vi "WILT Process Cycle Data.vi"(7 "WILT Summary Input":T1[](array[typedef]), 9 "Inverter File Headers":string[](array[string]), 10 "File Locations":T2[](array[typedef]), 11 "New File":bool[](array[boolean])) -> (2 "Units to Process":bool[](array[boolean]), 3 "WILT Summary Output":T1[](array[typedef]))   [LabVIEW 2016]
uses:
  Utility/Save File/File Setup (Public)/Type Definition/Save File DOE File Path Control.ctl
  Utility/Save File/File Setup (Public)/Type Definition/Save File DOE Data Save Filepaths.ctl
  Type Definitions/WILT Summary Data.ctl
  Utility/Save File/File Setup.lvlib
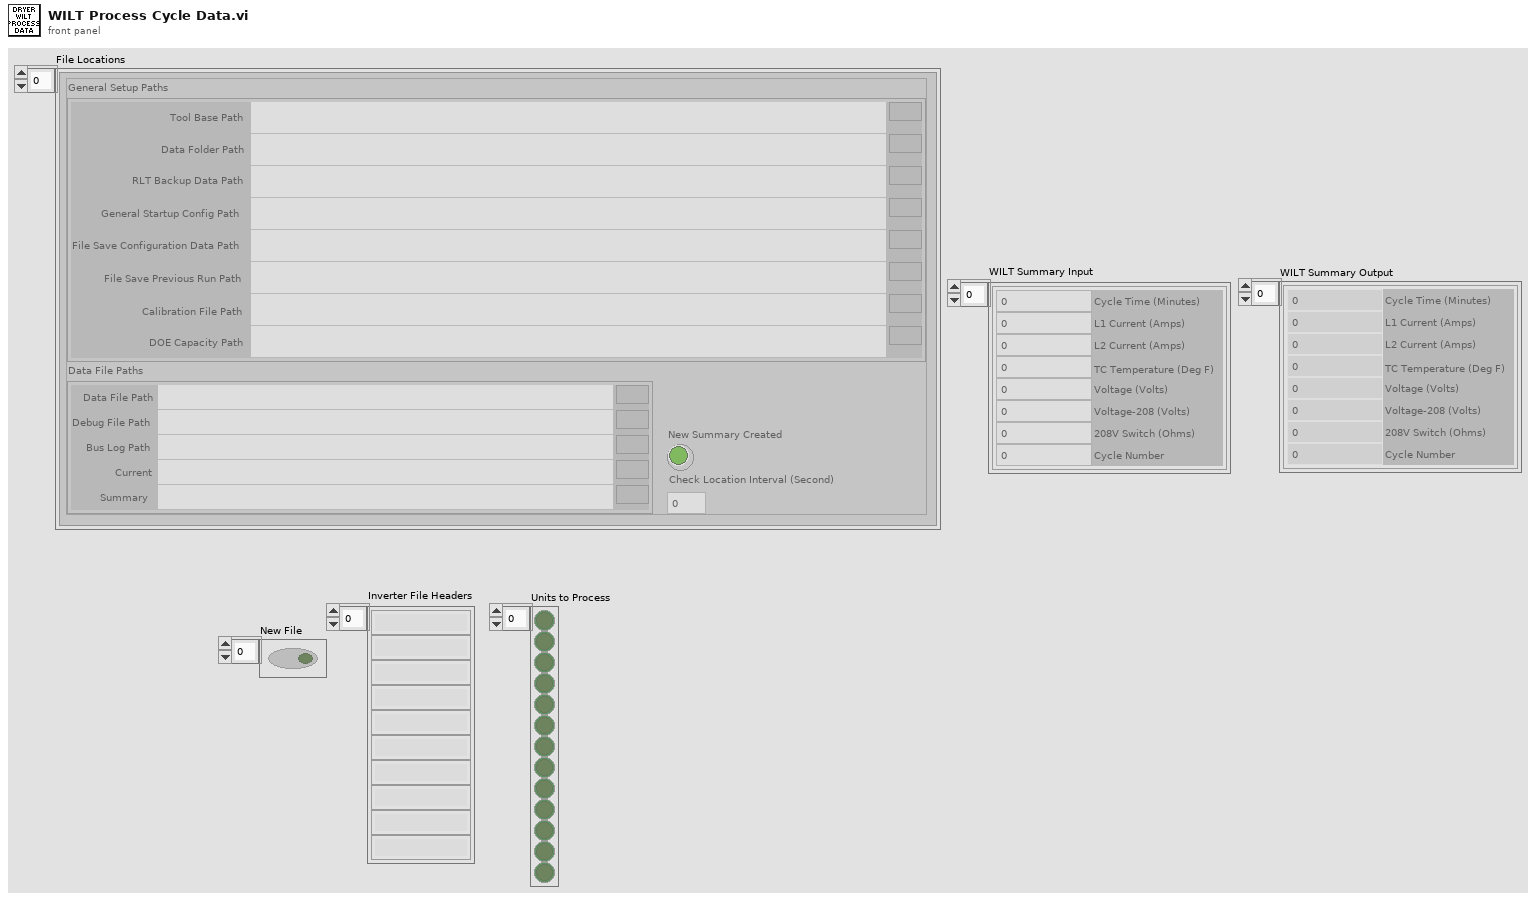
[diagram p1: front panel]
types:
  T1 = typedef "WILT Summary Data.ctl" = cluster{"Cycle Time (Minutes)":dbl, "L1 Current (Amps)":dbl, "L2 Current (Amps)":dbl, "TC Temperature (Deg F)":dbl, "Voltage (Volts)":dbl, "Voltage-208 (Volts)":dbl, "208V Switch (Ohms)":dbl, "Cycle Number":i32}
  T2 = typedef "File Setup.lvlib/Save File DOE File Path Control.ctl" = cluster{"General Setup Paths":cluster{"Calibration File Path":path, "DOE Capacity Path":path, "Data Folder Path":path, "RLT Backup Data Path":path, "Tool Base Path":path, "General Startup Config Path":path, "File Save Previous Run Path":path, "File Save Configuration Data Path":path}, "Data File Paths":T3, "New Summary Created":bool, "Check Location Interval (Second)":i32}
  T3 = typedef "File Setup.lvlib/Save File DOE Data Save Filepaths.ctl" = cluster{"Data File Path":path, "Debug File Path":path, "Bus Log Path":path, "Current":path, "Summary":path}
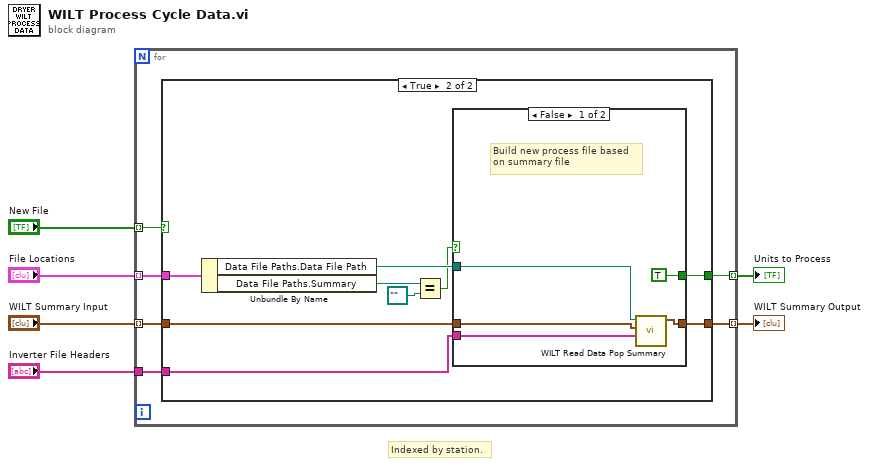
[diagram p0: block diagram]
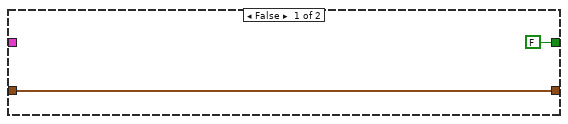
[diagram p2: hidden frame]
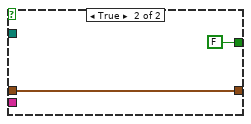
[diagram p3: hidden frame]
diagram:
  # "Indexed by station."
  n1 = for {
    tunnel: "New File" -> [w12] mode=indexing
    tunnel: "File Locations" -> [w11] mode=indexing
    tunnel: "Inverter File Headers" -> [w10]
    tunnel: [w9] -> w3 mode=indexing
    tunnel: [w8] -> w2 mode=indexing
    tunnel: "WILT Summary Input" -> [w7] mode=indexing
    n2 = case shown="True" w12 {
      tunnel: w11 -> [_ w23]
      tunnel: w10 -> [_ w21]
      tunnel: [w13 w20] -> w9
      tunnel: [FALSE w16] -> w8
      tunnel: w7 -> [w13 w15]
      frame False {
      }
      frame True {
        n3 = Unbundle By Name(w23) -> ("Data File Paths.Data File Path"=w22:path, "Data File Paths.Summary"=w19:path)
        n4 = Equal?(x=w19, y=path "") -> (x = y?=w17:bool)
        n5 = case shown="False" w17 {
          tunnel: w22 -> [w28 _]
          tunnel: w21 -> [w27 _]
          tunnel: [w26 w29] -> w20
          tunnel: [TRUE FALSE] -> w16
          tunnel: w15 -> [w24 w29]
          frame False {
            # "Build new process file based\non summary file"
            n6 = call "WILT Read Data Pop Summary.vi"("Inverter File Headers"=w27, "WILT Summary Cluster Input in"=w24, "Log Inverter File"=w28) -> ("WILT Summary Cluster Input out"=w26:T1)  [unwired: 8 in]
          }
          frame True {
          }
        }
      }
    }
  }
  "WILT Summary Output" <- w3
  "Units to Process" <- w2
